vi "ShortcutMenu.vi"(8 "error in":errorcluster, 9 "menu ref in":refnum<k9>, 11 "node in":refnum<class "My System.lvclass">) -> (0 "error out":errorcluster, 1 "menu ref out":refnum<k9>, 3 "node out":refnum<class "My System.lvclass">)   [LabVIEW 2014, in "My System.lvclass"]
doc: "Defines the behavior of the shortcut menu of the node."
uses:
  My System.lvclass
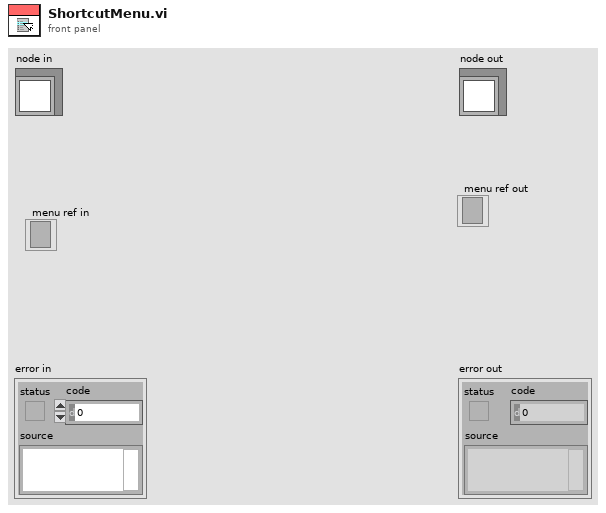
[diagram p1: front panel]
types:
  T1 = typedef "NISE_CEF_Node.lvclass/SubNodeCluster.ctl" = cluster{"subnodes menu name":string[], "subnodes class":string[]}
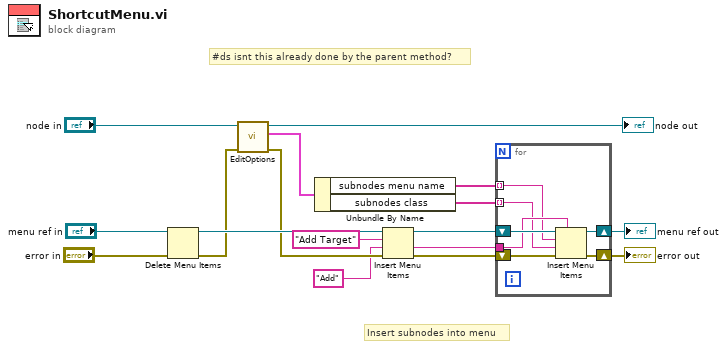
[diagram p0: block diagram]
diagram:
  # "#ds isnt this already done by the parent method?"
  # "Insert subnodes into menu"
  n1 = Delete Menu Items(6:"error in", 9:"menu ref in") -> (0:w15:errorcluster, 3:w16:refnum<k9>)  [unwired: 2 in]
  n2 = call-dynamic "EditOptions.vi"("error in"=w15, "node in"="node in") -> ("error out"=w10:errorcluster, "subnodes class"=w11:T1, "node out"=→"node out":refnum<class "My System.lvclass">)  [unwired: 6 in, 1 out]
  n3 = Unbundle By Name(w11) -> ("subnodes menu name"=w9:string[], "subnodes class"=w8:string[])
  n4 = Insert Menu Items(6:w10, 7:"Add" ("item tags"), 8:"Add Target", 9:w16) -> (0:w14:errorcluster, 1:w12:string, 3:w13:refnum<k9>)  [unwired: 2 in]
  n5 = for {
    shift-right: [w24] -> w4
    shift-left: w14 -> [w23]
    shift-right: [w21] -> w5
    shift-left: w13 -> [w22]
    tunnel: w12 -> [w20]
    tunnel: w9 -> [w19] mode=indexing
    tunnel: w8 -> [w18] mode=indexing
    n6 = Insert Menu Items(5:w20, 6:w23, 7:w18, 8:w19, 9:w22) -> (0:w24:errorcluster, 3:w21:refnum<k9>)  [unwired: 1 in, 1 out]
  }
  "error out" <- w4
  "menu ref out" <- w5
